vi "Init.vi"(8 "error in (no error)":errorcluster, 10 "Channel":i16=-10, 11 "AcquistionObject in":refnum<class "AcquistionObject.lvclass">) -> (0 "error out":errorcluster, 3 "AcquistionObject out":refnum<class "AcquistionObject.lvclass">)   [LabVIEW 2014, in "AcquisitionCoreObjects.lvlib" / "AcquistionObject.lvclass"]
uses:
  AcquistionObject.lvclass
  <vilib>/Utility/config.llb/NI_LVConfig.lvlib
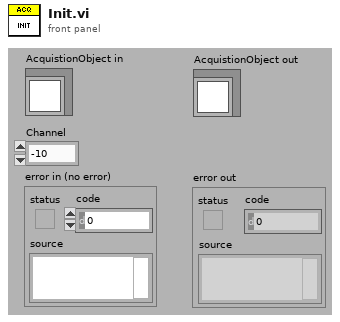
[diagram p1: front panel]
types:
  T1 = typedef "NI_LVConfig.lvlib/Config Data RefNum.ctl" = refnum<k1>
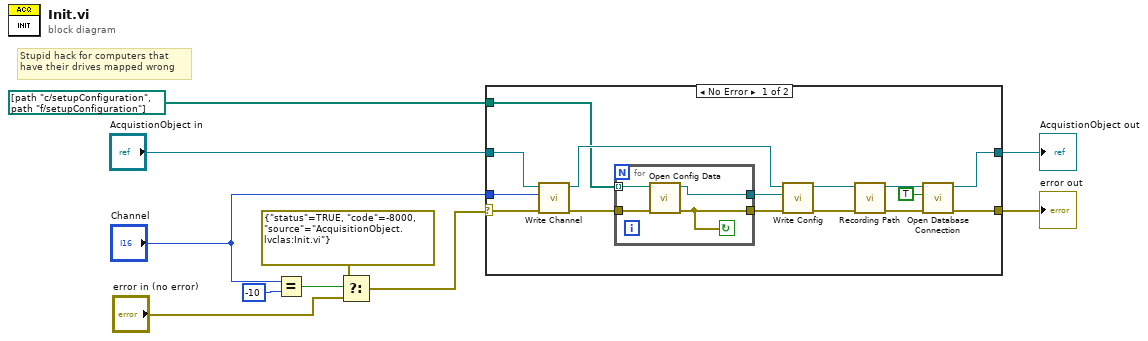
[diagram p0: block diagram]
diagram:
  # "Stupid hack for computers that \nhave their drives mapped wrong"
  n1 = Equal?(x="Channel", y=i16 -10 ("x")) -> (x = y?=w5:bool)
  n2 = Select(t=errorcluster {"status"=TRUE, "code"=-8000, "source"="AcquisitionObject.lvclas:Init.vi"}, s=w5, f="error in (no error)") -> (s? t:f=w3:errorcluster)
  n3 = case shown="No Error" w3 {
    selector: w3 -> [w17 w31]
    tunnel: [w12 w31] -> w10
    tunnel: [w13 w30] -> w8
    tunnel: "AcquistionObject in" -> [w23 w30]
    tunnel: path[] [path "c:/setupConfiguration", path "f:/setupConfiguration"] -> [w16 _]
    tunnel: "Channel" -> [w18 _]
    frame No Error {
      n4 = call-dynamic "Write Channel.vi"("error in (no error)"=w17, "Channel"=w18, "AcquistionObject in"=w23) -> ("error out"=w22:errorcluster, "AcquistionObject out"=w20:refnum<class "AcquistionObject.lvclass">)  [unwired: 7 in]
      n5 = for {
        tunnel: w22 -> [w29]
        tunnel: [w28] -> w25
        tunnel: [w26] -> w24
        tunnel: w16 -> [w27] mode=indexing
        stop <- w26 continue-if-true
        n6 = call <vilib>:"Open Config Data.vi"("error in (no error)"=w29, "configuration file path"=w27) -> ("error out"=w26:errorcluster, "refnum"=w28:T1)  [unwired: 7 in, 1 out]
      }
      n7 = call-dynamic "Write Config.vi"("error in (no error)"=w24, "config data"=w25, "AcquistionObject in"=w20) -> ("error out"=w21:errorcluster, "AcquistionObject out"=w19:refnum<class "AcquistionObject.lvclass">)  [unwired: 7 in]
      n8 = call-dynamic "Recording Path.vi"("error in (no error)"=w21, "AcquistionObject in"=w19) -> ("error out"=w14:errorcluster, "AcquistionObject out"=w15:refnum<class "AcquistionObject.lvclass">)  [unwired: 7 in, 1 out]
      n9 = call-dynamic "Open Database Connection.vi"("error in (no error)"=w14, "Initialize DatabaseQueue"=TRUE, "AcquistionObject in"=w15) -> ("error out"=w12:errorcluster, "AcquistionObject out"=w13:refnum<class "AcquistionObject.lvclass">)  [unwired: 7 in]
    }
    frame Error {
    }
  }
  "error out" <- w10
  "AcquistionObject out" <- w8
